vi "pharosTriggersGenerate.vi"(1 "off at the end":bool=TRUE) -> (0 "triggers":u8[](array[numeric]))   [LabVIEW 2017]
uses:
  globalUtilities.vi
panel:
  out "size(s)":i32
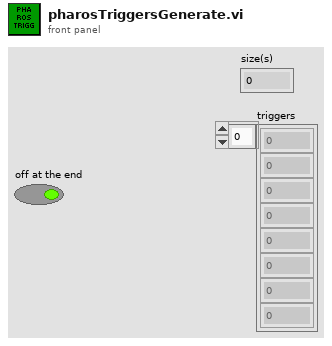
[diagram p1: front panel]
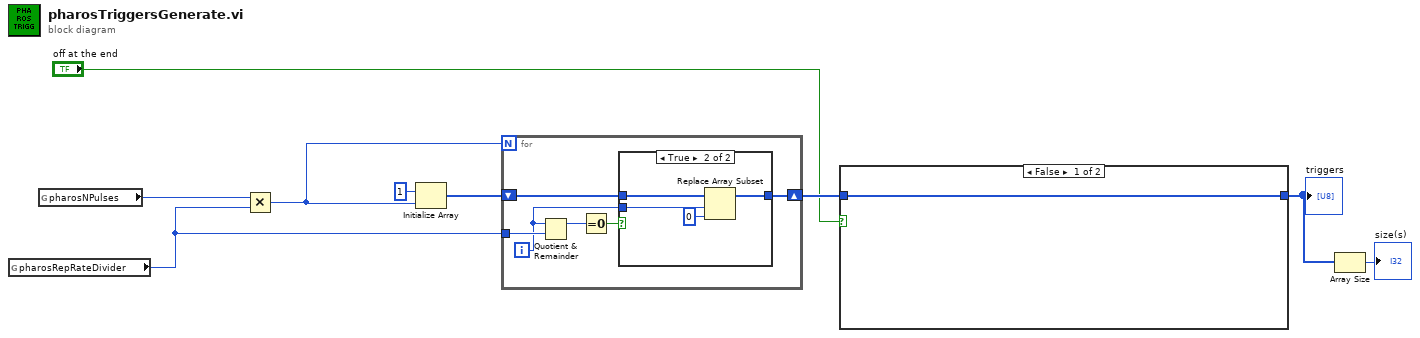
[diagram p0: block diagram]
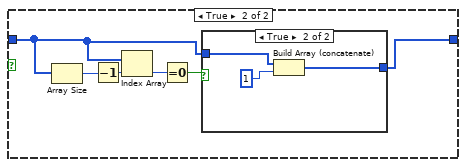
[diagram p2: hidden frame]
diagram:
  n1 = global read "globalUtilities.vi" "pharosRepRateDivider"() -> (w7:i32)
  n2 = global read "globalUtilities.vi" "pharosNPulses"() -> (w6:i32)
  n3 = Multiply(x=w6, y=w7) -> (x*y=w5:i32)
  n4 = Initialize Array(u8 1 ("element"), w5) -> (w8:u8[])
  n5 = for {
    N: w5 -> [_]
    tunnel: w7 -> [w14]
    shift-right: [w10] -> w4
    shift-left: w8 -> [w15]
    i -> [w11]
    n6 = Quotient & Remainder(x=w11, y=w14) -> (x-y*floor(x/y)=w13:i32)  [unwired: 1 out]
    n7 = Equal To 0?(x=w13) -> (x = 0?=w12:bool)
    n8 = case shown="True" w12 {
      tunnel: w15 -> [w16 w20]
      tunnel: w11 -> [_ w19]
      tunnel: [w16 w17] -> w10
      frame False {
      }
      frame True {
        n9 = Replace Array Subset(array=w20, new element=u8 0 ("new element/subarray"), index=w19) -> (w17:u8[])
      }
    }
  }
  n10 = case shown="False" "off at the end" {
    tunnel: w4 -> [w21 w24]
    tunnel: [w21 w23] -> w2
    frame False {
    }
    frame True {
      n11 = Array Size(array=w24) -> (size(s)=w25:i32)
      n12 = Decrement(x=w25) -> (x-1=w22:i32)
      n13 = Index Array(array=w24, index=w22) -> (element=w27:u8)
      n14 = Equal To 0?(x=w27) -> (x = 0?=w26:bool)
      n15 = case shown="True" w26 {
        tunnel: w24 -> [w28 w31]
        tunnel: [w28 w29] -> w23
        frame False {
        }
        frame True {
          n16 = Build Array (concatenate)(w31, u8 1) -> (w29:u8[])
        }
      }
    }
  }
  "triggers" <- w2
  n17 = Array Size(array=w2) -> (size(s)=→"size(s)":i32)
